vi "UDCWriteSetting.vi"(8 "Error In":errorcluster, 9 "value":string, 10 "name":string, 11 "clientId":string) -> (0 "Error Out":errorcluster)   [LabVIEW 2020, in "niceiplib.lvlib"]
doc: "UDC_SYMBOLS void UDCWriteSetting(const char *clientId, const char *name, const char *value);\n\nThis API is used to write back the CEIP settings."
uses:
  <vilib>/UDC/niceiplib.lvlib
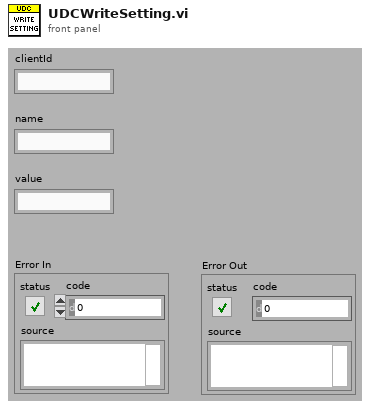
[diagram p1: front panel]
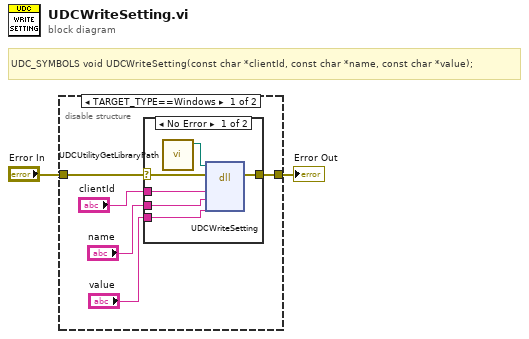
[diagram p0: block diagram]
diagram:
  # "UDC_SYMBOLS void UDCWriteSetting(const char *clientId, const char *name, const char *value);"
  n1 = disable-structure shown="TARGET_TYPE==Windows" {
    disable-tunnel: [w4 w15] -> w2
    disable-tunnel: "Error In" -> [w3 w15]
    frame condition #0 (active) {
      n2 = case shown="No Error" w3 {
        selector: w3 -> [w9 w14]
        tunnel: "clientId" -> [w13 _]
        tunnel: "name" -> [w12 _]
        tunnel: "value" -> [w11 _]
        tunnel: [w10 w14] -> w4
        frame No Error {
          n3 = call <vilib>:"UDCUtilityGetLibraryPath.vi"() -> ("Library Path"=w8:path)  [unwired: 11 in]
          n4 = dll-call lib="C:/2013LabVIEWCode/dist/vi.lib/UDC/niceiplib.*" fn="UDCWriteSetting"(path in=w8, error in=w9, "clientId"=w13, "name"=w12, "value"=w11) -> (error out=w10:errorcluster)  [unwired: 5 in, 1 out]
        }
        frame Error {
        }
      }
    }
    frame condition #1 {
    }
  }
  "Error Out" <- w2
